vi "RSZVB Define Group Of All Measured Ports.vi"(7 "Ports":i32[](array[numeric])=[1, 0, 0, 0, 0], 8 "error in (no error)":errorcluster {"code" format="%.0x"}, 9 "Group (1)":i32=1, 10 "Channel (1)":i32=1, 11 "VISA session":refnum<visa-resource-name>) -> (0 "error out":errorcluster {"code" format="%.0x"}, 3 "dup VISA session":refnum<visa-resource-name>)   [LabVIEW 2011]
doc: "This VI defines a port group numbered <group_no> containing an arbitrary selection of logical ports. The ports do not have to be numbered continuously (as for port groups defined via SOURce<Ch>:GROup<group_no>). \n\nNote(s):\n\n(1) It is not possible to create more than one port group with arbitrary ports. To avoid errors, use the setting command only while the channel contains a single port group (e.g. after a *RST). You can use the query to read out the ports for an arbitrary number of port groups created via SOURce<Ch>:GROup<group_no>.\n\nRemote-control command(s):\nSOURce<Ch>:GROup<group_no>:PORTs <log_port1>{,<log_port2> ...}"
uses:
  _utility/RSZVB Global Data.vi
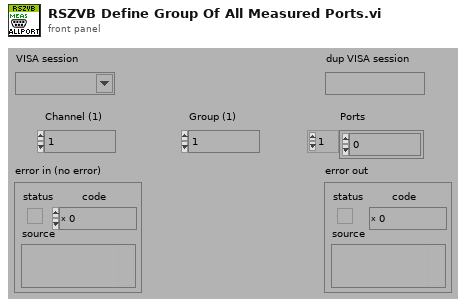
[diagram p1: front panel]
types:
  T1 = cluster{"Error Checking (T: On)":bool, "Installed Options":string[], "Data Valid?":bool, "Ports":i32, "Model":string[], "Option Checking (T: On)":bool}[]
  T2 = cluster{"Error Checking (T: On)":bool, "Installed Options":string[], "Data Valid?":bool, "Ports":i32, "Model":string[], "Option Checking (T: On)":bool}
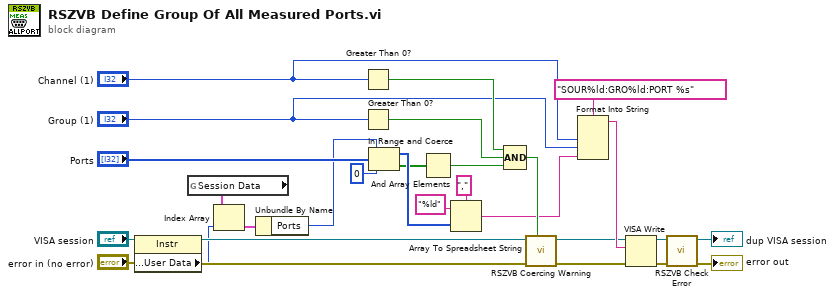
[diagram p0: block diagram]
diagram:
  n1 = property class="Instr"(reference="VISA session", error in="error in (no error)") -> (reference out=w29:refnum<visa-resource-name>, error out=w28:errorcluster, "General Settings:User Data"=w27:u32)
  n2 = global read "RSZVB Global Data.vi" "Session Data"() -> (w26:T1)
  n3 = Index Array(array=w26, index=w27) -> (element=w25:T2)
  n4 = Unbundle By Name(w25) -> ("Ports"=w2:i32)
  n5 = Greater Than 0?(x="Channel (1)") -> (x > 0?=w24:bool)
  n6 = Greater Than 0?(x="Group (1)") -> (x > 0?=w23:bool)
  n7 = In Range and Coerce(upper limit=w2, x="Ports", lower limit=0) -> (coerced(x)=w5:i32[], In Range?=w4:bool[])
  n8 = And Array Elements(Boolean array=w4) -> (logical AND=w3:bool)
  n9 = Array To Spreadsheet String(delimiter (Tab)=",", array=w5, 3:"%ld") -> (spreadsheet string=w11:string)
  n10 = Compound Arithmetic op=AND(w24, w23, w3) -> (w21:bool)
  n11 = call "RSZVB Coercing Warning.vi"("In Range?"=w21, "error in (no error)"=w28, "VISA session"=w29) -> ("error out"=w18:errorcluster, "dup VISA session"=w17:refnum<visa-resource-name>)  [unwired: 7 in]
  n12 = Format Into String(format string="SOUR%ld:GRO%ld:PORT %s", "Channel (1)", "Group (1)", w11) -> (resulting string=w22:string)  [unwired: 2 in, 1 out]
  n13 = VISA Write(VISA resource name=w17, write buffer=w22, error in (no error)=w18) -> (VISA resource name out=w20:refnum<visa-resource-name>, error out=w19:errorcluster)  [unwired: 1 out]
  n14 = call "RSZVB Check Error.vi"("error in (no error)"=w19, "VISA session"=w20) -> ("error out"=→"error out":errorcluster, "dup VISA session"=→"dup VISA session":refnum<visa-resource-name>)  [unwired: 8 in]
